vi "vel calc C1 (express VI).vi"(8 "error in":errorcluster, 10 "Action":T1) -> (0 "error out":errorcluster, 1 "dt":i32, 2 "dx":i32, 3 "dx/dt":dbl, 5 "Counter Value":i32)   [LabVIEW 2017]
uses:
  Action Items.ctl
  <vilib>/myRIO/Common/Instrument Driver Framework/myRIO v1.0/Encoder/typedefs/Encoder Signal Mode.ctl
  <vilib>/myRIO/Instrument Drivers/Onboard IO/Encoder/typedefs/Encoder Reference.ctl
  <vilib>/myRIO/Common/Instrument Driver Framework/Utilities/typedefs/myRIO Generic Hardware Reference.ctl
  <vilib>/myRIO/Common/Instrument Driver Framework/Utilities/typedefs/Hardware Version Enum.ctl
  <vilib>/myRIO/Common/Instrument Driver Framework/Utilities/typedefs/myRIO v1.0 Reference.ctl
  <vilib>/myRIO/Common/Instrument Driver Framework/Utilities/typedefs/Generic FPGA Reference.ctl
  <vilib>/myRIO/Common/Instrument Driver Framework/myRIO v1.0/Encoder/typedefs/Encoder Channels Enum.ctl
  <vilib>/myRIO/Common/Instrument Driver Framework/myRIO v1.0/Encoder/typedefs/Encoder Configuration v1.0.ctl
  <vilib>/userdefined/High Color/nirio_resource_hc.ctl
  <vilib>/myRIO/Common/Instrument Driver Framework/Utilities/vis/Is FPGA Ref Available.vi
  <vilib>/myRIO/Common/Instrument Driver Framework/myRIO v1.0/Encoder/vis/myRIO v1.1 Open Encoder.vi
  <vilib>/myRIO/Instrument Drivers/Onboard IO/Encoder/vis/Read.vi
  <vilib>/myRIO/Common/Instrument Driver Framework/Utilities/vis/Validate Channels.vi
  <vilib>/myRIO/Common/Instrument Driver Framework/myRIO v1.0/Encoder/vis/myRIO v1.0 Reserve Encoder.vi
  <vilib>/myRIO/Common/Instrument Driver Framework/myRIO v1.0/Encoder/vis/myRIO v1.0 Build MUX Configuration Encoder.vi
  <vilib>/myRIO/Common/Instrument Driver Framework/myRIO v1.0/Resource Manager/vis/myRIO v1.0 Reserve Channel List.vi
  <vilib>/myRIO/Common/Instrument Driver Framework/myRIO v1.0/Resource Manager/vis/myRIO v1.0 Create Configuration List.vi
  <vilib>/myRIO/Common/Instrument Driver Framework/myRIO v1.0/Resource Manager/vis/myRIO v1.0 Reserve Channel.vi
  <vilib>/myRIO/Common/Instrument Driver Framework/myRIO v1.0/Resource Manager/vis/myRIO v1.0 Unreserve Channel.vi
  <vilib>/myRIO/Common/Instrument Driver Framework/myRIO v1.0/Resource Manager/vis/myRIO v1.0 Build Mutex Name.vi
  <vilib>/functionblocks/Counter/Elapsed Timer/Elapsed Timer.vi
  <vilib>/Utility/VariantDataType/GetNumericInfo.vi
  <vilib>/Utility/error.llb/Error Cluster From Error Code.vi
  <vilib>/myRIO/Common/Instrument Driver Framework/myRIO v1.0/myRIO v1.1 Open.vi
  <vilib>/myRIO/Common/Instrument Driver Framework/Utilities/vis/IO Manager.vi
  <vilib>/myRIO/Common/Instrument Driver Framework/Utilities/vis/Configuration Manager.vi
  <vilib>/myRIO/Common/Instrument Driver Framework/myRIO v1.0/Resource Manager/vis/myRIO v1.0 Configure IO.vi
  <vilib>/myRIO/Common/Instrument Driver Framework/myRIO v1.0/myRIO v1.0 Close.vi
  <vilib>/myRIO/Common/Instrument Driver Framework/myRIO v1.0/Encoder/vis/myRIO v1.0 Configure Encoder.vi
  <vilib>/myRIO/Common/Instrument Driver Framework/myRIO v1.0/Encoder/vis/myRIO v1.0 Read Encoder.vi
  <vilib>/functionblocks/FB Core/FB Core.xnode
  <vilib>/myRIO/Express VI/Onboard IO/Encoder/Encoder Express VI.xnode
  <vilib>/myRIO/Instrument Drivers/Onboard IO/Encoder/vis/myRIO Encoder Open.xnode
  <vilib>/myRIO/Common/Instrument Driver Framework/myRIO v1.0/Encoder/typedefs/Encoder Count Direction Enum.ctl
  <vilib>/functionblocks/NI_FunctionBlock Libraries.lvlib
  <vilib>/myRIO/Instrument Drivers/Onboard IO/Encoder/Encoder.lvlib
panel:
  out "elapsed time (ms)":i32
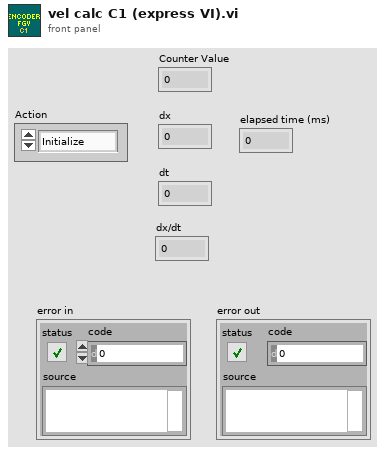
[diagram p1: front panel]
types:
  T1 = typedef "Action Items.ctl" = enum16{"Initialize", "Read"}
  T2 = typedef "Encoder.lvlib/Encoder Reference.ctl" = cluster{"myRIO Reference":T3, "Encoder Channels Enum":T7}
  T3 = typedef "myRIO Generic Hardware Reference.ctl" = cluster{"myRIO Model":T4, "myRIO Hardware Reference":T5}
  T4 = typedef "Hardware Version Enum.ctl" = enum16{"Unknown", "myRIO-1900", "myRIO-1950", "roboRIO", "NI ELVIS RIO CM"}
  T5 = typedef "myRIO v1.0 Reference.ctl" = cluster{"Generic FPGA Reference":T6, "Allow multiple opens":bool}
  T6 = typedef "Generic FPGA Reference.ctl" = refnum<k20>
  T7 = typedef "Encoder Channels Enum.ctl" = enum16{"Not Connected", "C/ENC0", "C/ENC1", "A/ENC", "B/ENC", "DIO/ENC0", "DIO/ENC1", "DIO/ENC2", "DIO/ENC3", "DIO/ENC4"}
  T8 = typedef "Encoder Signal Mode.ctl" = enum16{"Quadrature phase signal", "Step and direction signal"}
  T9 = typedef "nirio_resource_hc.ctl" = tag
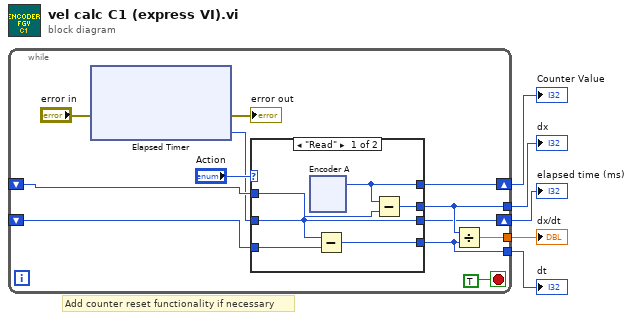
[diagram p0: block diagram]
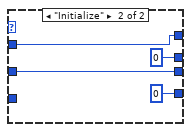
[diagram p2: hidden frame]
diagram:
  # "Add counter reset functionality if necessary"
  n1 = while {
    shift-right: [w10] -> w1
    shift-left: _ -> [w9]
    shift-right: [w15] -> w3
    shift-left: _ -> [w16]
    tunnel: [w13] -> w4
    tunnel: [w12] -> w5
    tunnel: [w11] -> w2
    stop <- TRUE stop-if-true
    n2 = xnode "Elapsed Timer"("error in"="error in") -> ("error out"=→"error out":errorcluster, "elapsed time (ms)"=w6:i32)
    n3 = case shown="\"Read\"" "Action" {
      tunnel: w16 -> [w59 w109]
      tunnel: [w54 w109] -> w15
      tunnel: [w58 0] -> w13
      tunnel: [w57 0] -> w12
      tunnel: [w56 w106] -> w10
      tunnel: w6 -> [w56 w106]
      tunnel: w9 -> [w55 _]
      frame "Read" {
        n4 = xnode "Encoder A"() -> ("Counter Value"=w54:i32)  [unwired: 2 in, 3 out]
        n5 = Subtract(x=w56, y=w55) -> (x-y=w57:i32)
        n6 = Subtract(x=w54, y=w59) -> (x-y=w58:i32)
      }
      frame "Initialize" {
      }
    }
    n7 = Divide(x=w13, y=w12) -> (x/y=w11:dbl)
  }
  "Counter Value" <- w3
  "dx" <- w4
  "dt" <- w5
  "dx/dt" <- w2
  "elapsed time (ms)" <- w1
